vi "Function.vi"(8 "error in (no error)":errorcluster, 9 "Numeric B":T1, 10 "Numeric A":T1, 11 "Subtract in":refnum<class "Subtract_CPLX_DBL.lvclass">) -> (0 "error out":errorcluster, 2 "Result":T1, 3 "Subtract out":refnum<class "Subtract_CPLX_DBL.lvclass">)   [LabVIEW 2021, in "Subtract_CPLX_DBL.lvclass"]
uses:
  Subtract_CPLX_DBL.lvclass
  Type.ctl
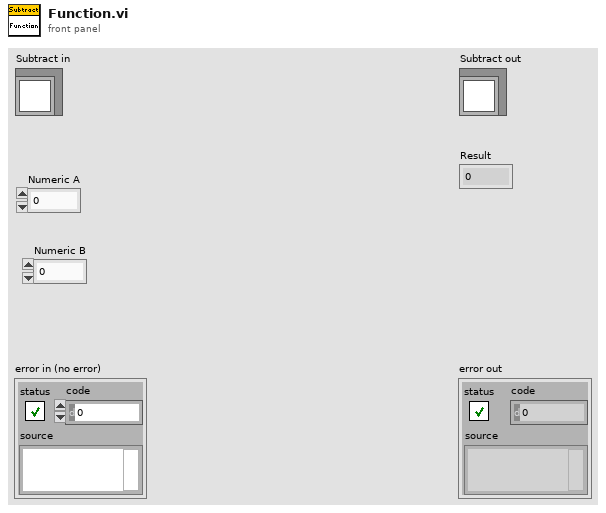
[diagram p1: front panel]
types:
  T1 = typedef "Subtract_CPLX_DBL.lvclass/Type.ctl" = cdb
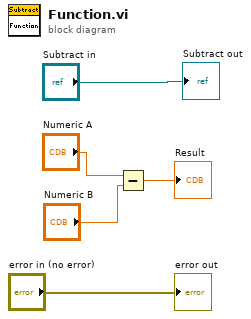
[diagram p0: block diagram]
diagram:
  n1 = Subtract(x="Numeric A", y="Numeric B") -> (x-y=→"Result":T1)
  "error out" <- "error in (no error)"
  "Subtract out" <- "Subtract in"
